vi "PresureGetSubVI.vi"(0 "COM in":refnum<visa-resource-name>="COM5", 1 "Fehler (Eingang)":errorcluster) -> (6 "Status Gauge#1":i32(ring) items=["data OK", "underrange", "overrange", "sensor error", "sensor off", "no sensor", "ID error"], 8 "Status Gauge#2":i32(ring) items=["data OK", "underrange", "overrange", "sensor error", "sensor off", "no sensor", "ID error"], 10 "COM out":refnum<visa-resource-name>, 14 "Pressure Gauge#1":dbl format="%.3e", 15 "Pressure Gauge#2":dbl format="%.3e", 16 "Cluster (Ausgang)":errorcluster)   [LabVIEW 2013]
uses:
  Argos0v7/Dependencies/Pfeiffer TPG261+262 Single+Dual Gauge/Dual Gauge.lvlib
panel:
  # "mbar"
  # "mbar"
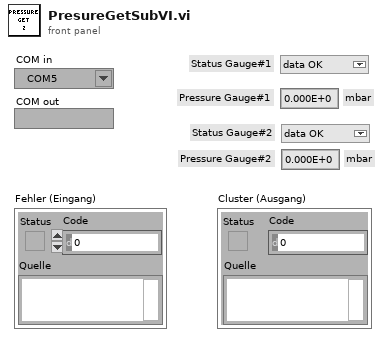
[diagram p1: front panel]
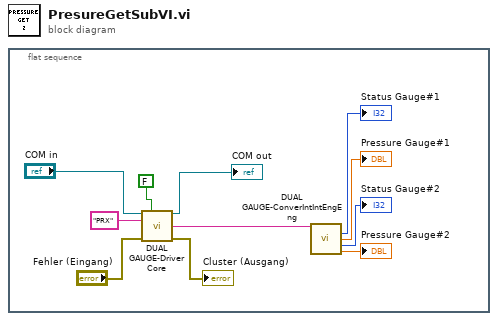
[diagram p0: block diagram]
diagram:
  n1 = flat-sequence {
    frame #0 {
      n2 = call "DUAL GAUGE-Driver Core.vi"("Referenz in"="COM in", "Write/Read"=FALSE, "Command"="PRX", "Fehler (Eingang)"="Fehler (Eingang)") -> ("Referenz out"=→"COM out":refnum<visa-resource-name>, "String Out"=w8:string, "Cluster (Ausgang)"=→"Cluster (Ausgang)":errorcluster)  [unwired: 9 in]
      n3 = call "DUAL GAUGE-ConverIntIntEngEng.vi"("String in"=w8) -> ("Integer1 out"=→"Status Gauge#1":u8, "Eng1 out"=→"Pressure Gauge#1":dbl, "Integer2 out"=→"Status Gauge#2":u8, "Eng2 out"=→"Pressure Gauge#2":dbl)  [unwired: 11 in]
    }
  }
